vi "AB_Engine_Get_AppShell.vi"(8 "error in (no error)":errorcluster, 10 "useBCRTE":bool, 11 "useFFRTE":bool) -> (0 "error out":errorcluster, 3 "pathAppShell":path)   [LabVIEW 2020]
uses:
  <resource>/Framework/Providers/Common/provcom_StringGlobals.vi
  <vilib>/AppBuilder/AB_Classes/Application/AB_Application.lvclass
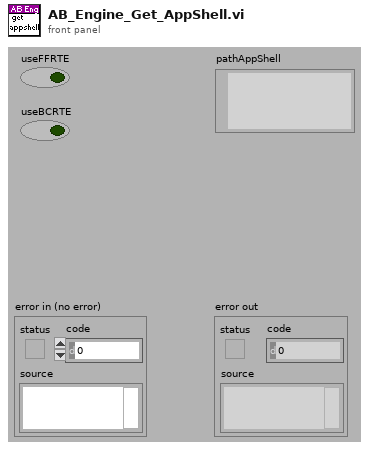
[diagram p1: front panel]
types:
  T1 = enum32{"invalid OS target", "Mac OS", "Windows 3.1", "Windows 95/NT", "Solaris 1", "Solaris 2", "HP-UX", "PowerMAX", "Linux", "Irix", "Rhapsody", "BeOS", "AIX", "OSF1", "VxWorks", "PharLap", "Carbon", "RTX", "Windows x64", "Linux x64", "Mac OS X x64"}
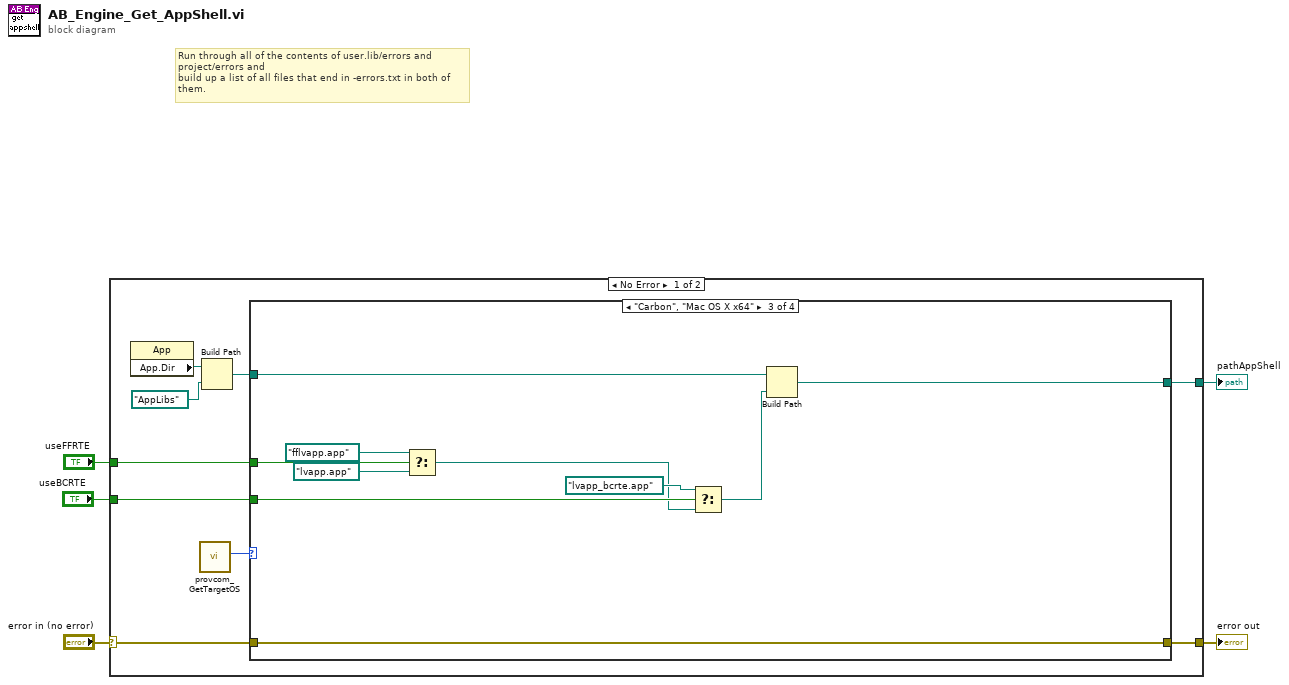
[diagram p0: block diagram]
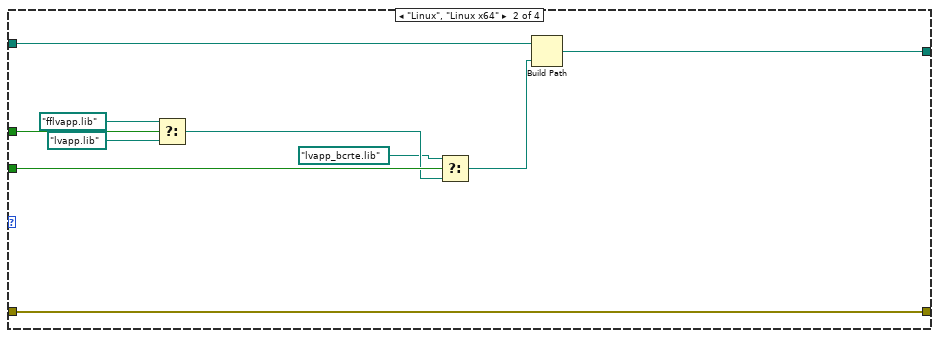
[diagram p3: hidden frame]
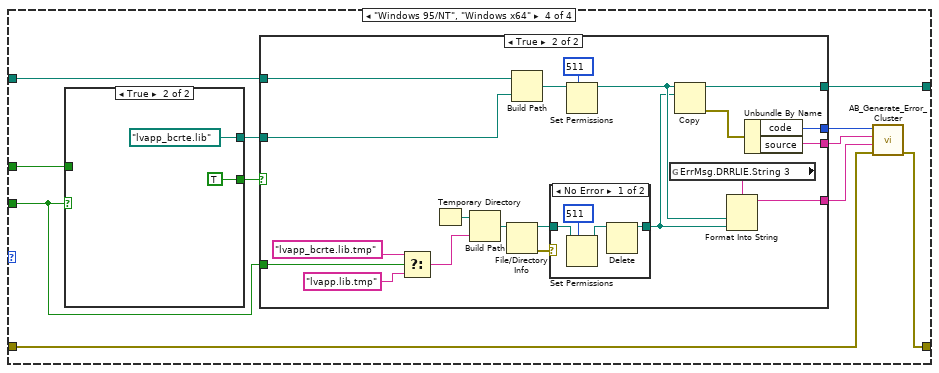
[diagram p4: hidden frame]
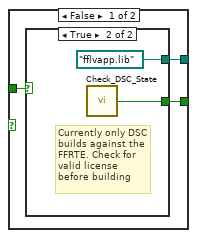
[diagram p5: hidden frame]
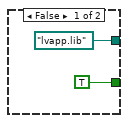
[diagram p6: hidden frame]
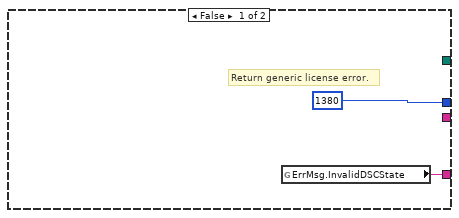
[diagram p7: hidden frame]
diagram:
  # "Run through all of the contents of user.lib/errors and project/errors and\nbuild up a list of all files that end in -errors.txt in both of them."
  n1 = case shown="No Error" "error in (no error)" {
    selector: "error in (no error)" -> [w11 w83]
    tunnel: [w9 w83] -> w4
    tunnel: "useFFRTE" -> [w10 _]
    tunnel: [w8 _] -> w2
    tunnel: "useBCRTE" -> [w6 _]
    frame No Error {
      n2 = property class="App"() -> ("App.Dir"=w13:path)  [unwired: 2 in, 2 out]
      n3 = call <resource>:"provcom_GetTargetOS.vi"() -> ("App.TargetOS"=w7:T1)  [unwired: 11 out]
      n4 = Build Path(base path=w13, name or relative path=path "AppLibs") -> (appended path=w12:path)
      n5 = case shown="\"Carbon\", \"Mac OS X x64\"" w7 {
        tunnel: [_ w20 w33 w41] -> w8
        tunnel: w11 -> [w15 w25 w30 w43]
        tunnel: [w15 w25 w30 w40] -> w9
        tunnel: w12 -> [_ w22 w35 w42]
        tunnel: w10 -> [_ w21 w34 w39]
        tunnel: w6 -> [_ w19 w28 w36]
        frame Default {
        }
        frame "Linux", "Linux x64" {
          n6 = Select(t=path "fflvapp.lib", s=w21, f=path "lvapp.lib") -> (s? t:f=w18:path)
          n7 = Select(t=path "lvapp_bcrte.lib", s=w19, f=w18) -> (s? t:f=w17:path)
          n8 = Build Path(base path=w22, name or relative path=w17) -> (appended path=w20:path)
        }
        frame "Carbon", "Mac OS X x64" {
          n9 = Select(t=path "fflvapp.app", s=w34, f=path "lvapp.app") -> (s? t:f=w27:path)
          n10 = Select(t=path "lvapp_bcrte.app", s=w28, f=w27) -> (s? t:f=w26:path)
          n11 = Build Path(base path=w35, name or relative path=w26) -> (appended path=w33:path)
        }
        frame "Windows 95/NT", "Windows x64" {
          n12 = case shown="True" w36 {
            tunnel: w39 -> [w49 _]
            tunnel: [w48 path "lvapp_bcrte.lib"] -> w38
            tunnel: [w47 TRUE ("active")] -> w37
            frame False {
              n13 = case shown="True" w49 {
                tunnel: [path "lvapp.lib" path "fflvapp.lib"] -> w48
                tunnel: [TRUE w52] -> w47
                frame False {
                }
                frame True {
                  # "Currently only DSC builds against the FFRTE. Check for valid license before building"
                  n14 = call <vilib>:"Check_DSC_State.vi"() -> ("active"=w52:bool)  [unwired: 1 out]
                }
              }
            }
            frame True {
            }
          }
          n15 = case shown="True" w37 {
            tunnel: [1380 ("code") w77] -> w46
            tunnel: [_ w76] -> w45
            tunnel: [w56 w75] -> w44
            tunnel: w42 -> [_ w73]
            tunnel: [_ w72] -> w41
            tunnel: w38 -> [_ w62]
            tunnel: w36 -> [_ w61]
            frame False {
              # "Return generic license error."
              n16 = global read "provcom_StringGlobals.vi" "ErrMsg.InvalidDSCState"() -> (w56:string)
            }
            frame True {
              n17 = Select(t="lvapp_bcrte.lib.tmp" ("name or relative path"), s=w61, f="lvapp.lib.tmp" ("name or relative path")) -> (s? t:f=w59:string)
              n18 = Temporary Directory() -> (w65:path)
              n19 = Build Path(base path=w65, name or relative path=w59) -> (appended path=w66:path)
              n20 = File/Directory Info(path=w66) -> (path out=w68:path, error out=w67:errorcluster)  [unwired: 1 in, 5 out]
              n21 = Build Path(base path=w73, name or relative path=w62) -> (appended path=w70:path)
              n22 = case shown="No Error" w67 {
                tunnel: w68 -> [w80 w82]
                tunnel: [w81 w82] -> w64
                frame No Error {
                  n23 = Set Permissions(7:i16 511 ("permissions"), 11:w80) -> (3:w79:path)  [unwired: 1 in, 3 out]
                  n24 = Delete(path (use dialog)=w79) -> (deleted path=w81:path)  [unwired: 1 in, 5 out]
                }
                frame Error {
                }
              }
              n25 = Set Permissions(7:i16 511 ("permissions"), 11:w70) -> (3:w69:path)  [unwired: 1 in, 3 out]
              n26 = global read "provcom_StringGlobals.vi" "ErrMsg.DRRLIE.String 3"() -> (w63:string)
              n27 = Copy(10:w64, 11:w69) -> (0:w74:errorcluster, 3:w72:path)  [unwired: 1 in, 3 out]
              n28 = Format Into String(format string=w63, w69, w64) -> (resulting string=w75:string)  [unwired: 2 in, 1 out]
              n29 = Unbundle By Name(w74) -> ("code"=w77:i32, "source"=w76:string)
            }
          }
          n30 = call <vilib>:"AB_Generate_Error_Cluster.vi"("error in (no error)"=w43, "Additional Message"=w44, "source"=w45, "Code"=w46) -> ("error out"=w40:errorcluster)  [unwired: 7 out]
        }
      }
    }
    frame Error {
    }
  }
  "error out" <- w4
  "pathAppShell" <- w2
